vi "Configure Transform Precoding.vi"(6 "Enabled (On)":bool=TRUE, 7 "BWP (BWP0)":i32(ring) items=["BWP0"], 8 "error in (no error)":errorcluster, 9 "CC (1)":T1=1, 10 "Instance (1)":T2=1, 11 "VISA resource name":refnum<visa-resource-name>) -> (0 "error out":errorcluster, 3 "VISA resource name out":refnum<visa-resource-name>)   [LabVIEW 2020, in "Rohde&Schwarz CMWXP NR FR1 Measurement.lvlib"]
doc: "Specifies whether the <BWP> on carrier <no> uses a transform precoding VI.\n\nAttribute:\nRSCMWXPNRFR1M_ATTR_TRANSFORM_PRECODING\n\nRemote-control command:\nCONFigure:NRSub:MEAS<i>[:CC<no>]:BWPart:PUSCh:DFTPrecoding"
uses:
  <instrlib>/Rohde&Schwarz CMWXP NR FR1 Measurement/Rohde&Schwarz CMWXP NR FR1 Measurement.lvlib
  <instrlib>/Rohde&Schwarz CMWXP NR FR1 Measurement/Private/_Instance.ctl
  <instrlib>/Rohde&Schwarz CMWXP NR FR1 Measurement/Private/_Carrier Component.ctl
  <instrlib>/Rohde&Schwarz CMWXP NR FR1 Measurement/Private/rsidr_core.llb/rsidr_core.lvlib
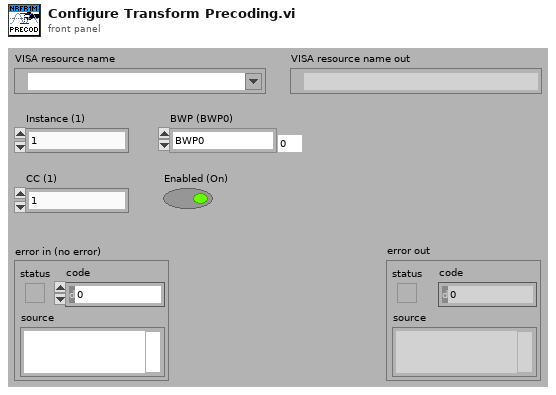
[diagram p1: front panel]
types:
  T1 = typedef "Rohde&Schwarz CMWXP NR FR1 Measurement.lvlib/_Carrier Component.ctl" = i32
  T2 = typedef "Rohde&Schwarz CMWXP NR FR1 Measurement.lvlib/_Instance.ctl" = i32
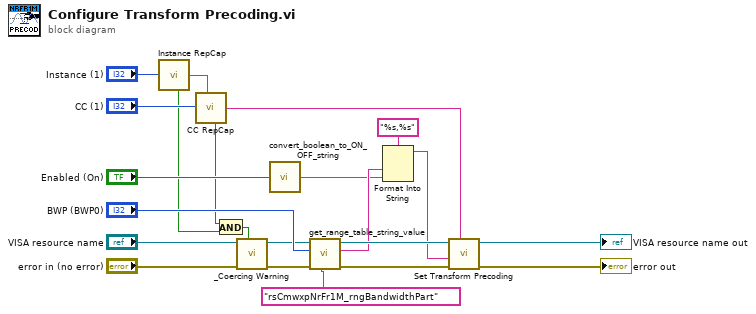
[diagram p0: block diagram]
diagram:
  n1 = call <instrlib>:"Instance RepCap.vi"("Instance In"="Instance (1)") -> ("In Range?"=w1:bool, "RepCap Identifier Out"=w17:string)  [unwired: 1 in]
  n2 = call <instrlib>:"CC RepCap.vi"("CC In"="CC (1)", "RepCap String In (\"\")"=w17) -> ("In Range?"=w2:bool, "RepCap Identifier Out"=w14:string)
  n3 = And(x=w2, y=w1) -> (x .and. y?=w3:bool)
  n4 = call <instrlib>:"_Coercing Warning.vi"("In Range?"=w3, "error in (no error)"="error in (no error)", "VISA resource name"="VISA resource name") -> ("error out"=w5:errorcluster, "VISA resource name out"=w4:refnum<visa-resource-name>)  [unwired: 7 in]
  n5 = call <instrlib>:"convert_boolean_to_ON_OFF_string.vi"("boolean value in"="Enabled (On)") -> ("string value out"=w9:string)  [unwired: 4 in]
  n6 = call <instrlib>:"get_range_table_string_value.vi"("Range Table ID in"="rsCmwxpNrFr1M_rngBandwidthPart", "error in"=w5, "I32 input"="BWP (BWP0)", "VISA resource name"=w4) -> ("error out"=w19:errorcluster, "String Value out"=w10:string, "VISA resource name out"=w18:refnum<visa-resource-name>)  [unwired: 5 in]
  n7 = Format Into String(format string="%s,%s", w10, w9) -> (resulting string=w8:string)  [unwired: 2 in, 1 out]
  n8 = call "Set Transform Precoding"("Repeated Capabilities"=w14, "error in (no error)"=w19, "Transform Precoding ()"=w8, "instrument handle"=w18) -> ("error out"=→"error out":errorcluster, "instrument handle out"=→"VISA resource name out":refnum<visa-resource-name>)  [unwired: 6 in]
